vi "Form Endpoint.vi"(10 "Endpoint":string, 11 "Resource":string) -> (3 "Resource/Endpoint":string)   [LabVIEW 2020, in "Routing and Faulting System Explorer.lvlib"]
uses:
  Routing and Faulting System Explorer.lvlib
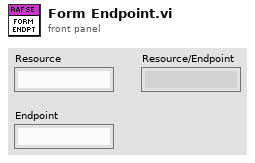
[diagram p1: front panel]
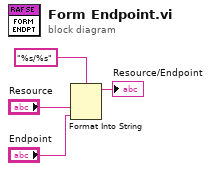
[diagram p0: block diagram]
diagram:
  n1 = Format Into String(format string="%s/%s", "Resource", "Endpoint") -> (resulting string=→"Resource/Endpoint":string)  [unwired: 2 in, 1 out]
